vi "NF87XX.get status.vi"(0 "i ref in":refnum<vi>, 5 "error in (no error)":errorcluster) -> (14 "i ref out":refnum<vi>, 16 "status":string, 19 "error out":errorcluster)   [LabVIEW 2014, in "NF87XX.lvlib"]
doc: "Returns the status to the device.\n\nauthor: Stefan Götte\ndata: 09-JAN-2007\n\n\nLicense Agreement for this software:\n\nCopyright (C)\nGesellschaft für Schwerionenforschung, GSI\nPlanckstr. 1\n64291 Darmstadt\nGermany\n\nContact: D.Beck@gsi.de \n\nThis program is free software; you can redistribute it and/or modify it under the terms of the GNU General Public License as published by the Free Software Foundation; either version 2 of the license, or (at your option) any later version.\n\nThis program is distributed in the hope that it will be useful, but WITHOUT ANY WARRANTY; without even the implied warranty of MERCHANTABILITY or FITNESS FOR A PARTICULAR PURPOSE. See the GNU General License for more details (http://www.gnu.org).\n\nGesellschaft für Schwerionenforschung, GSI\nPlanckstr. 1, 64291 Darmstadt, Germany\nFor all questions and ideas contact: M.Richter@gsi.de, H.Brand@gsi.de or D.Beck@gsi.de.\nLast update: 17-JUN-2004"
uses:
  NF87XX.lvlib
  CS_PHELIX/PH_Basics/PH_StatusHandler/PH_StatusHandler.Status.ctl
  CS_PHELIX/PH_Basics/PH_StatusHandler/PH_StatusHandler.lvlib
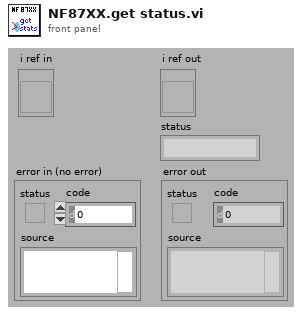
[diagram p1: front panel]
types:
  T1 = typedef "PH_StatusHandler.lvlib/PH_StatusHandler.Status.ctl" = i16
  T2 = enum16{"User....", "DEF", "DIAG", "INI", "LOCK", "UNLOCK", "MAP", "SAV", "VER", "ACC", "CHL", "FOR", "GO", "HAL", "MOF", "MON", "MPV", "POS", "REL", "REV", "STA", "STO", "TYP", "VEL", "ABS", "SER", "NOS", "DRT", "FLI", "RLI", "FIN", "RIN", "AIN", "IN", "JOF", "JON", "OUT", "RES FINE", "RES COARSE", "02 (HEX)", "PWM", "CNT", "TMR", "HOSTNAME", "IPADDR", "IPMODE", "NETMASK", "GATEWAY", "DNSSRVR", "PASSWD", "ECHO", "MACADDR"}
  T3 = typedef "NF87XX.lvlib/NF87XX.i attribute.ctl" = cluster{"Con Settings":T4, "Drivers":T5[], "Status":cluster{"Service ID":i32, "Status":T1}, "Joystick available":bool, "VISA Resource":string}
  T4 = typedef "NewFocusPico - Driver np.lvlib/VISA & TCPIP Control.ctl" = cluster{"VISA or TCP/IP":bool, "Init Connection":bool, "Close Connection":bool, "Resource Name":refnum<visa-resource-name>, "hostname":string, "connection ID":refnum<k5>}
  T5 = typedef "NF87XX.lvlib/NF87XX.driver Settings.ctl" = cluster{"Name":string, "Driver Type":T6, "Pico Parameter type":T7, "Acceleration [Steps/s²]":cluster{"Motor 0":dbl, "Motor 1":dbl, "Motor 2":dbl}, "Start Velocity [Steps/s]":cluster{"Motor 0":dbl, "Motor 1":dbl, "Motor 2":dbl}, "Velocity [Steps/s]":cluster{"Motor 0":dbl, "Motor 1":dbl, "Motor 2":dbl}, "axis channel":i32, "Position":i32, "Position Service ID":i32}
  T6 = typedef "NF87XX.lvlib/NF87XX.driver Type.ctl" = enum16{"not defined", "3-ch open loop drv", "1-ch closed loop drv"}
  T7 = typedef "NewFocusPico - Driver np.lvlib/Pico Parameters.ctl" = cluster{"Pico Type":enum16{"Open-Loop Pico", "Close-Loop Pico", "Pico Ultra"}, "Acceleration (steps/sec^2)":string, "Velocity ( Hz)":string, "Driver":string, "Motor":string, "Channel":string, "Process Step":string}
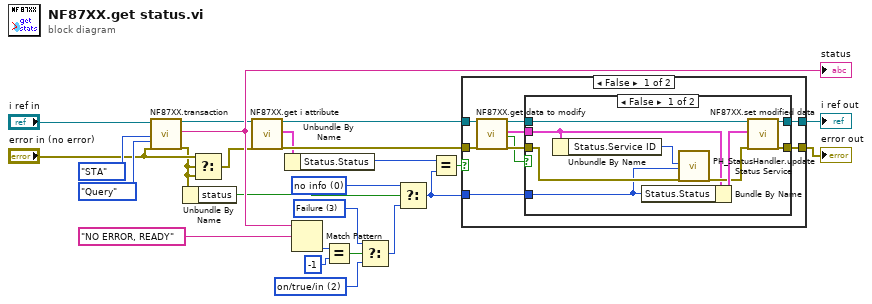
[diagram p0: block diagram]
diagram:
  w2 = T1 0 items=["no info", "off/false/out", "on/true/in", "Failure", "Alarm", "Status 1", "Status 2", "Status 3"] ("t")
  w9 = T1 2 items=["no info", "off/false/out", "on/true/in", "Failure", "Alarm", "Status 1", "Status 2", "Status 3"] ("f")
  w10 = T1 3 items=["no info", "off/false/out", "on/true/in", "Failure", "Alarm", "Status 1", "Status 2", "Status 3"] ("Status.Status")
  n1 = call "NF87XX.transaction.vi"("i ref in"="i ref in", "MCL Cmd"=T2."STA", "Query/Set"=enum16{"Query", "Set"}."Query", "error in (no error)"="error in (no error)") -> ("i ref out"=w18:refnum<vi>, "Read String"=w22:string, "error out"=w6:errorcluster)  [unwired: 13 in]
  "status" <- w22
  n2 = Unbundle By Name(w6) -> ("status"=w5:bool)
  n3 = Select(t="error in (no error)", s=w6, f=w6) -> (s? t:f=w7:errorcluster)
  n4 = call "NF87XX.get i attribute.vi"("i ref in"=w18, "error in (no error)"=w7) -> ("i ref out"=w17:refnum<vi>, "i attribute"=w13:T3, "error out"=w16:errorcluster)  [unwired: 15 in]
  n5 = Unbundle By Name(w13) -> ("Status.Status"=w8:T1)
  n6 = Match Pattern(string=w22, regular expression="NO ERROR, READY") -> (offset past match=w15:i32)  [unwired: 1 in, 3 out]
  n7 = Equal?(x=w15, y=-1) -> (x = y?=w11:bool)
  n8 = Select(t=w10, s=w11, f=w9) -> (s? t:f=w3:T1)
  n9 = Select(t=w2, s=w5, f=w3) -> (s? t:f=w1:T1)
  n10 = Equal?(x=w8, y=w1) -> (x = y?=w4:bool)
  n11 = case shown="False" w4 {
    tunnel: [w32 w47] -> w20
    tunnel: [w31 w46] -> w19
    tunnel: w17 -> [w30 w47]
    tunnel: w16 -> [w29 w46]
    tunnel: w1 -> [w26 _]
    frame False {
      n12 = call "NF87XX.get data to modify.vi"("i ref in"=w30, "error in (no error)"=w29) -> ("i ref out"=w33:refnum<vi>, "i attribute"=w28:T3, "timed out"=w27:bool, "error out"=w34:errorcluster)  [unwired: 14 in]
      n13 = case shown="False" w27 {
        tunnel: w34 -> [w39 w44]
        tunnel: w33 -> [w43 w45]
        tunnel: [w42 w45] -> w32
        tunnel: [w41 w44] -> w31
        tunnel: w28 -> [w37 _]
        tunnel: w26 -> [w35 _]
        frame False {
          n14 = Unbundle By Name(w37) -> ("Status.Service ID"=w36:i32)
          n15 = Bundle By Name(cluster=w37, "Status.Status"=w35) -> (w40:T3)
          n16 = call "PH_StatusHandler.update Status Service.vi"("Service ID"=w36, "Status"=w35, "error in (no error)"=w39) -> ("error out"=w38:errorcluster)  [unwired: 16 in]
          n17 = call "NF87XX.set modified data.vi"("i ref in"=w43, "i attribute"=w40, "error in (no error)"=w38) -> ("i ref out"=w42:refnum<vi>, "error out"=w41:errorcluster)  [unwired: 15 in]
        }
        frame True {
        }
      }
    }
    frame True {
    }
  }
  "error out" <- w19
  "i ref out" <- w20
